vi "Number To Digits.vi"(0 "Value":i32) -> (1 "Digits":i8[](array[numeric]), 2 "Num Digits":i32)   [LabVIEW 2025]
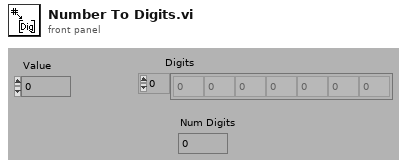
[diagram p1: front panel]
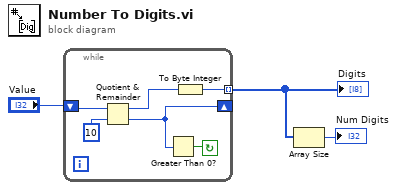
[diagram p0: block diagram]
diagram:
  n1 = while {
    tunnel: [w4] -> w1 mode=indexing
    shift-left: "Value" -> [w8]
    shift-right: [w6] -> _
    stop <- w7 continue-if-true
    n2 = Quotient & Remainder(x=w8, y=10) -> (x-y*floor(x/y)=w5:i32, floor(x/y)=w6:i32)
    n3 = Greater Than 0?(x=w6) -> (x > 0?=w7:bool)
    n4 = To Byte Integer(number=w5) -> (8bit integer=w4:i8)
  }
  "Digits" <- w1
  n5 = Array Size(array=w1) -> (size(s)=→"Num Digits":i32)
